vi "Read scopes.vi"(8 "error in (no error)":errorcluster, 11 "Oauth2 in":refnum<class "Oauth2.lvclass">) -> (0 "error out":errorcluster, 2 "scopes":string[](array[string]), 3 "Oauth2 out":refnum<class "Oauth2.lvclass">)   [LabVIEW 2020, in "Oauth2.lvclass"]
uses:
  Oauth2.lvclass
  Oauth2.lvclass/Oauth2.ctl
  OAuthToken/OAuth2 Token Element -- enum.ctl
  OAuthToken/OAuthAccessToken.lvclass
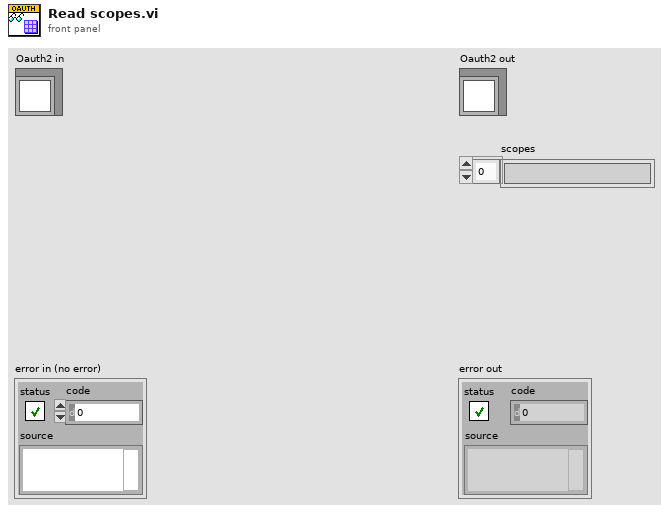
[diagram p1: front panel]
types:
  T1 = typedef "OAuthAccessToken.lvclass/OAuth2 Token Element -- enum.ctl" = enum16{"client_id", "client_secret", "response_type", "scope", "redirect_uri", "error", "error_description", "error_uri", "grant_type", "code", "access_token", "token_type", "expires_in", "username", "password", "refresh_token", "code_challenge", "code_challenge_method", "reverse_proxy_uri", "endpoint element"}
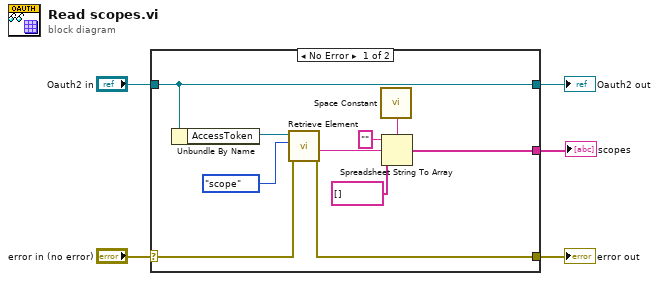
[diagram p0: block diagram]
diagram:
  n1 = case shown="No Error" "error in (no error)" {
    selector: "error in (no error)" -> [w12 w16]
    tunnel: [w11 w16] -> w2
    tunnel: [w15 w17] -> w3
    tunnel: "Oauth2 in" -> [w15 w17]
    tunnel: [w6 _] -> w1
    frame No Error {
      n2 = Unbundle By Name(w15) -> ("AccessToken"=w14:refnum<class "OAuthAccessToken.lvclass">)
      n3 = call "Retrieve Element.vi"("error in (no error)"=w12, "Token element"=OAuth2_Token_Element_--_enum."scope", "OAuthAccessToken in"=w14) -> ("error out"=w11:errorcluster, "Value"=w10:string)  [unwired: 4 in, 3 out]
      n4 = call <vilib>:"Space Constant.vi"() -> ("String"=w9:string)
      n5 = Spreadsheet String To Array(delimiter (Tab)=w9, format string="", spreadsheet string=w10, array type (2D Dbl)=string[] [] ("scopes")) -> (array=w6:string[])
    }
    frame Error {
    }
  }
  "error out" <- w2
  "Oauth2 out" <- w3
  "scopes" <- w1
